vi "MessageSender.vi"() -> ()   [LabVIEW 2018]
uses:
  <vilib>/myRIO/Instrument Drivers/Onboard IO/AO/typedefs/AO Reference.ctl
  <vilib>/myRIO/Common/Instrument Driver Framework/Utilities/typedefs/myRIO Generic Hardware Reference.ctl
  <vilib>/myRIO/Common/Instrument Driver Framework/Utilities/typedefs/Hardware Version Enum.ctl
  <vilib>/myRIO/Common/Instrument Driver Framework/Utilities/typedefs/myRIO v1.0 Reference.ctl
  <vilib>/myRIO/Common/Instrument Driver Framework/Utilities/typedefs/Generic FPGA Reference.ctl
  <vilib>/myRIO/Common/Instrument Driver Framework/myRIO v1.0/AO/typedefs/AO Channels List.ctl
  <vilib>/myRIO/Common/Instrument Driver Framework/myRIO v1.0/AO/typedefs/AO Channels Enum.ctl
  <vilib>/myRIO/Common/Instrument Driver Framework/Utilities/typedefs/Analog Scaling Constants List.ctl
  <vilib>/myRIO/Common/Instrument Driver Framework/Utilities/typedefs/Analog Scaling Constants.ctl
  <vilib>/userdefined/High Color/nirio_resource_hc.ctl
  <vilib>/myRIO/Common/Instrument Driver Framework/ELVIS III v1.0/AO/vis/ELVIS III v1.1 Open AO.vi
  <vilib>/myRIO/Common/Instrument Driver Framework/Utilities/vis/Validate Channels.vi
  <vilib>/myRIO/Common/Instrument Driver Framework/ELVIS III v1.0/AO/vis/ELVIS III v1.0 Reserve AO.vi
  <vilib>/myRIO/Common/Instrument Driver Framework/ELVIS III v1.0/AO/vis/ELVIS III v1.0 Close AO.vi
  <vilib>/myRIO/Common/Instrument Driver Framework/ELVIS III v1.0/AO/vis/ELVIS III v1.0 Build MUX Configuration AO.vi
  <vilib>/myRIO/Common/Instrument Driver Framework/ELVIS III v1.0/Resource Manager/vis/ELVIS III v1.0 Reserve Channel List.vi
  <vilib>/myRIO/Common/Instrument Driver Framework/ELVIS III v1.0/AO/vis/ELVIS III v1.0 Unreserve AO.vi
  <vilib>/myRIO/Common/Instrument Driver Framework/ELVIS III v1.0/Resource Manager/vis/ELVIS III v1.0 Reserve Channel.vi
  <vilib>/myRIO/Common/Instrument Driver Framework/ELVIS III v1.0/Resource Manager/vis/ELVIS III v1.0 Unreserve Channel.vi
  <vilib>/myRIO/Common/Instrument Driver Framework/ELVIS III v1.0/Resource Manager/vis/ELVIS III v1.0 Unreserve Channel List.vi
  <vilib>/myRIO/Common/Instrument Driver Framework/ELVIS III v1.0/Resource Manager/vis/ELVIS III v1.0 Build Mutex Name.vi
  <vilib>/Utility/VariantDataType/GetNumericInfo.vi
  <vilib>/Utility/error.llb/Error Cluster From Error Code.vi
  <vilib>/myRIO/Common/Instrument Driver Framework/ELVIS III v1.0/ELVIS III v1.1 Open.vi
  <vilib>/myRIO/Common/Instrument Driver Framework/Utilities/vis/IO Manager.vi
  <vilib>/myRIO/Common/Instrument Driver Framework/Utilities/vis/Configuration Manager.vi
  <vilib>/myRIO/Common/Instrument Driver Framework/myRIO v1.0/myRIO v1.0 Close.vi
  <vilib>/myRIO/Common/Instrument Driver Framework/ELVIS III v1.0/AO/vis/ELVIS III v1.0 Write AO.vi
  <vilib>/myRIO/Instrument Drivers/Onboard IO/AO/vis/myRIO AO Open.xnode
  <vilib>/myRIO/Instrument Drivers/Onboard IO/AO/AO.lvlib
panel:
  in  "Stop":bool
  in  "Input String":string
  in  "Send Message":bool
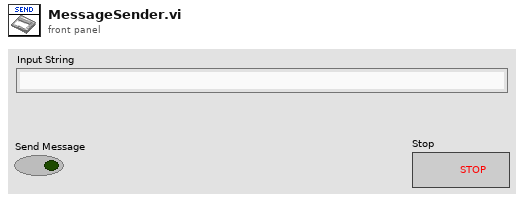
[diagram p1: front panel]
types:
  T1 = typedef "AO.lvlib/AO Reference.ctl" = cluster{"myRIO Reference":T2, "AO Channel List":T6, "AO Scaling Constant List":T8}
  T2 = typedef "myRIO Generic Hardware Reference.ctl" = cluster{"myRIO Model":T3, "myRIO Hardware Reference":T4}
  T3 = typedef "Hardware Version Enum.ctl" = enum16{"Unknown", "myRIO-1900", "myRIO-1950", "roboRIO", "NI ELVIS RIO CM", "ELVIS III"}
  T4 = typedef "myRIO v1.0 Reference.ctl" = cluster{"Generic FPGA Reference":T5, "Allow multiple opens":bool}
  T5 = typedef "Generic FPGA Reference.ctl" = refnum<k20>
  T6 = typedef "AO Channels List.ctl" = T7[]
  T7 = typedef "AO Channels Enum.ctl" = enum16{"Not Connected", "AudioOut/Left", "AudioOut/Right", "C/AO0", "C/AO1", "A/AO0", "A/AO1", "B/AO0", "B/AO1"}
  T8 = typedef "Analog Scaling Constants List.ctl" = T9[]
  T9 = typedef "Analog Scaling Constants.ctl" = cluster{"LSB Weight (Volts)":dbl, "Offset (Volts)":dbl, "Signed?":bool}
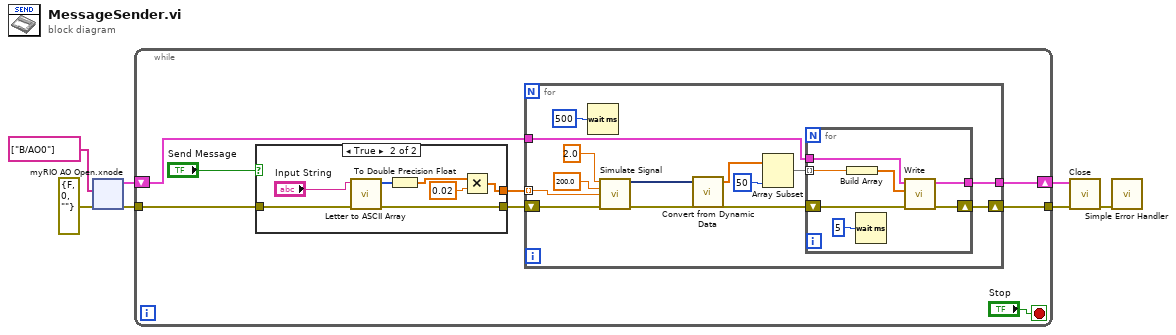
[diagram p0: block diagram]
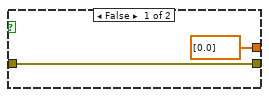
[diagram p2: hidden frame]
diagram:
  n1 = xnode "myRIO AO Open.xnode"("error in (no error)"=errorcluster {"status"=FALSE, "code"=0, "source"=""}, "Channel Names"=tag[] ["B/AO0"]) -> ("error out"=w7:errorcluster, "AO Ref Out"=w6:T1)  [unwired: 1 in]
  n2 = while {
    tunnel: [w14] -> w2
    shift-right: [w9] -> w3
    shift-left: w6 -> [w15]
    tunnel: w7 -> [w8]
    stop <- "Stop" stop-if-true
    n3 = case shown="True" "Send Message" {
      tunnel: [w16 w19] -> w12
      tunnel: [dbl[] [0.0] w18] -> w11
      tunnel: w8 -> [w16 w20]
      frame False {
      }
      frame True {
        n4 = call "Letter to ASCII Array.vi"("error in (no error)"=w20, "Input String"="Input String") -> ("error out"=w19:errorcluster, "String to ASCII Array"=w21:u8[])  [unwired: 8 in]
        n5 = To Double Precision Float(number=w21) -> (double precision float=w24:dbl[])
        n6 = Multiply(x=w24, y=0.02) -> (x*y=w18:dbl[])
      }
    }
    n7 = for {
      tunnel: w15 -> [w37]
      shift-right: [w35] -> w14
      shift-left: w12 -> [w30]
      tunnel: w11 -> [w27] mode=indexing
      tunnel: [w25] -> w9
      n8 = Wait (ms)(milliseconds to wait=u32 500) -> ()  [unwired: 1 out]
      n9 = call "Simulate Signal"("Offset"=2.0, "Frequency"=200.0, "Amplitude"=w27, "error in (no error)"=w30) -> ("Sine"=w36:dynamicdata, "error out"=w29:errorcluster)  [unwired: 10 in]
      n10 = call "Convert from Dynamic Data"("Dynamic Data Type"=w36) -> ("Array"=w33:dbl[])  [unwired: 3 in]
      n11 = Array Subset(array=w33, length=50) -> (w31:dbl[])  [unwired: 1 in]
      n12 = for {
        tunnel: w37 -> [w44]
        shift-right: [w40] -> w35
        shift-left: w29 -> [w43]
        tunnel: w31 -> [w42] mode=indexing
        tunnel: [w38] -> w25
        n13 = Build Array(w42) -> (w41:dbl[])
        n14 = Wait (ms)(milliseconds to wait=u32 5) -> ()  [unwired: 1 out]
        n15 = call <vilib>:"Write.vi"("error in (no error)"=w43, "Values"=w41, "AO Ref In"=w44) -> ("error out"=w40:errorcluster, "AO Ref Out"=w38:T1)  [unwired: 6 in]
      }
    }
  }
  n16 = call <vilib>:"Close.vi"("error in (no error)"=w2, "AO Ref In"=w3) -> ("error out"=w1:errorcluster)  [unwired: 9 in]
  n17 = call <vilib>:"Simple Error Handler.vi"("error in (no error)"=w1) -> ()  [unwired: 4 in, 5 out]
